vi "Created Aliases.vi"(11 "TEMPLATE Actor in":refnum<class "TEMPLATE Actor.lvclass">) -> (2 "Created Aliases":T1)   [LabVIEW 2020, in "_Template.lvlib" / "Templates.lvlib" / "TEMPLATE Actor.lvlib" / "TEMPLATE Actor.lvclass"]
uses:
  TEMPLATE Actor.lvclass
  jettl/jettl/Actor/Actor/Actor.lvclass
  jettl/jettl/Actor/Created Aliases.ctl
  jettl/jettl/Actor/Actor.lvlib
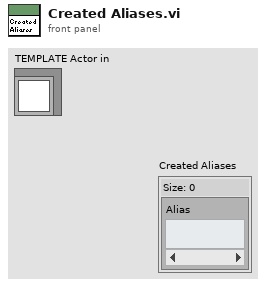
[diagram p1: front panel]
types:
  T1 = typedef "jettl.lvlib/Actor.lvlib/Created Aliases.ctl" = set{string}
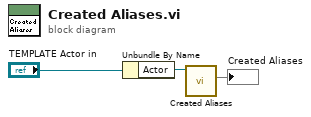
[diagram p0: block diagram]
diagram:
  n1 = Unbundle By Name("TEMPLATE Actor in") -> ("Actor"=w2:refnum<class "Actor.lvclass">)
  n2 = call-dynamic "Created Aliases.vi"("Actor in"=w2) -> ("Created Aliases"=→"Created Aliases":T1)  [unwired: 10 in]
